vi "get_x_iteration_values.vi"(8 "error in (no error)":errorcluster, 11 "TrajectoryAK101022Resonance in":refnum<class "TrajectoryAK101022Resonance.lvclass">) -> (0 "error out":errorcluster, 1 "fly-back offset [iterations]":u16, 2 "fly-forward offset [iterations]":u16, 3 "TrajectoryAK101022Resonance out":refnum<class "TrajectoryAK101022Resonance.lvclass">, 4 "iterations per pixel":u16, 5 "scan segment [iterations]":u16)   [LabVIEW 2010, in "TrajectoryAK101022Resonance.lvclass"]
uses:
  TrajectoryAK101022Resonance.lvclass
  FPGAWrapper/FPGAWrapperAK101022Resonance/FPGAWrapperAK101022Resonance/FPGAWrapperAK101022Resonance.lvclass
  TrajectoryAK101022Resonance.lvclass/TrajectoryAK101022Resonance.ctl
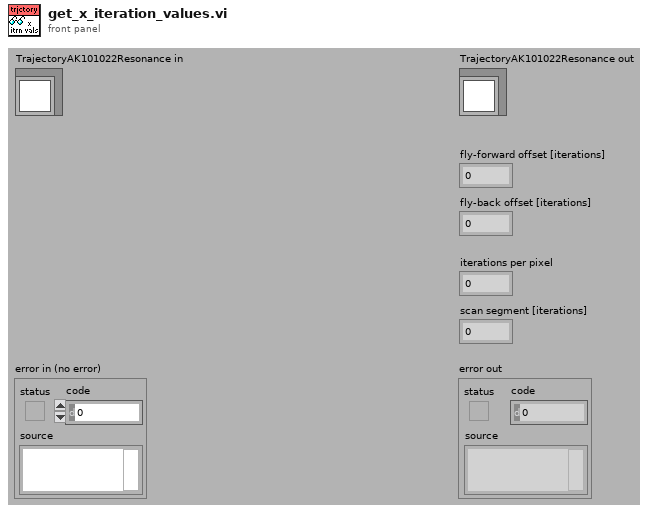
[diagram p1: front panel]
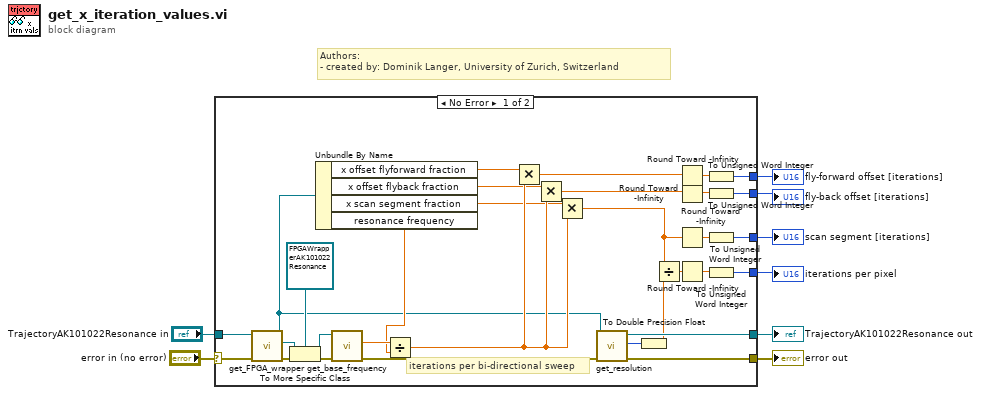
[diagram p0: block diagram]
diagram:
  # "Authors: \n- created by: Dominik Langer, University of Zurich, Switzerland"
  n1 = case shown="No Error" "error in (no error)" {
    selector: "error in (no error)" -> [w14 w41]
    tunnel: [w28 w41] -> w7
    tunnel: [w30 w40] -> w5
    tunnel: "TrajectoryAK101022Resonance in" -> [w13 w40]
    tunnel: [w35 _] -> w4
    tunnel: [w31 _] -> w3
    tunnel: [w20 _] -> w2
    tunnel: [w23 _] -> w1
    frame No Error {
      # "iterations per bi-directional sweep"
      n2 = call-dynamic "get_FPGA_wrapper.vi"("error in (no error)"=w14, "TrajectoryMG100122GenericFPGA in"=w13) -> ("error out"=w17:errorcluster, "GenericFPGAWrapper.lvclass"=w18:refnum<class "GenericFPGAWrapper.lvclass">, "TrajectoryMG100122GenericFPGA out"=w9:refnum<class "TrajectoryAK101022Resonance.lvclass">)  [unwired: 7 in]
      n3 = To More Specific Class(target class=refnum<class "FPGAWrapperAK101022Resonance.lvclass"> refnum ("FPGAWrapperAK101022Resonance.lvclass"), reference=w18, error in=w17) -> (specific class reference=w15:refnum<class "FPGAWrapperAK101022Resonance.lvclass">, error out=w16:errorcluster)
      n4 = Unbundle By Name(w9) -> ("x offset flyforward fraction"=w12:dbl, "x offset flyback fraction"=w11:dbl, "x scan segment fraction"=w10:dbl, "resonance frequency"=w38:dbl[unit])
      n5 = call "get_base_frequency.vi"("error in (no error)"=w16, "FPGAWrapperAK101022Resonance in"=w15) -> ("error out"=w29:errorcluster, "base frequency"=w39:dbl[unit])  [unwired: 7 in, 1 out]
      n6 = Divide(x=w39, y=w38) -> (x/y=w24:dbl)
      n7 = Multiply(x=w12, y=w24) -> (x*y=w37:dbl)
      n8 = Multiply(x=w11, y=w24) -> (x*y=w32:dbl)
      n9 = Multiply(x=w10, y=w24) -> (x*y=w21:dbl)
      n10 = call-dynamic "get_resolution.vi"("error in (no error)"=w29, "TrajectoryAK101022Resonance in"=w9) -> ("error out"=w28:errorcluster, "x resolution"=w27:i32, "TrajectoryAK101022Resonance out"=w30:refnum<class "TrajectoryAK101022Resonance.lvclass">)  [unwired: 6 in, 1 out]
      n11 = To Double Precision Float(number=w27) -> (double precision float=w26:dbl)
      n12 = Divide(x=w21, y=w26) -> (x/y=w25:dbl)
      n13 = Round Toward -Infinity(1:w37) -> (0:w36:dbl)
      n14 = Round Toward -Infinity(1:w32) -> (0:w34:dbl)
      n15 = Round Toward -Infinity(1:w21) -> (0:w22:dbl)
      n16 = Round Toward -Infinity(1:w25) -> (0:w33:dbl)
      n17 = To Unsigned Word Integer(number=w36) -> (unsigned 16bit integer=w35:u16)
      n18 = To Unsigned Word Integer(number=w34) -> (unsigned 16bit integer=w31:u16)
      n19 = To Unsigned Word Integer(number=w22) -> (unsigned 16bit integer=w23:u16)
      n20 = To Unsigned Word Integer(number=w33) -> (unsigned 16bit integer=w20:u16)
    }
    frame Error {
    }
  }
  "error out" <- w7
  "TrajectoryAK101022Resonance out" <- w5
  "fly-forward offset [iterations]" <- w4
  "fly-back offset [iterations]" <- w3
  "iterations per pixel" <- w2
  "scan segment [iterations]" <- w1
